vi "Calculate Torque.vi"() -> ()   [LabVIEW 2019]
doc: "This VI calculates the total torque resulting from two seperate force acting at two distinct moment arms. it uses a subvi to do the cross product.\n\nPK\nP3600"
uses:
  typedefs/torque vector.ctl
  P2 start/typedefs/moment arm vector.ctl
  P2 start/typedefs/force vector.ctl
panel:
  in  "Force B":T1={"Fx"=0.0, "Fy"=0.0, "Fz"=10.0}
  in  "Force A":T1={"Fx"=0.0, "Fy"=10.0, "Fz"=0.0}
  in  "Moment Arm B":T2={"Rx"=0.0, "Ry"=10.0, "Rz"=0.0}
  in  "Moment Arm A":T2={"Rx"=10.0, "Ry"=0.0, "Rz"=0.0}
  out "Resultant Torque":T3={"Nx"=100.0, "Ny"=0.0, "Nz"=100.0}
  # "Calculating Torques\n\nPK\nP3600"
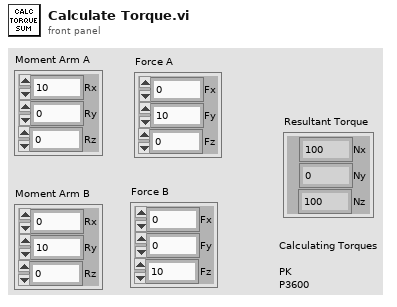
[diagram p1: front panel]
types:
  T1 = typedef "force vector.ctl" = cluster{"Fx":dbl, "Fy":dbl, "Fz":dbl}
  T2 = typedef "moment arm vector.ctl" = cluster{"Rx":dbl, "Ry":dbl, "Rz":dbl}
  T3 = typedef "torque vector.ctl" = cluster{"Nx":dbl, "Ny":dbl, "Nz":dbl}
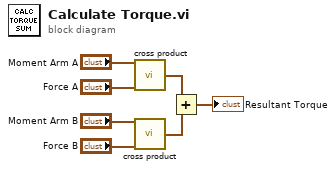
[diagram p0: block diagram]
diagram:
  n1 = call "cross product.vi"("Moment Arm"="Moment Arm A", "Force"="Force A") -> ("Torque"=w3:T3)  [unwired: 13 in]
  n2 = call "cross product.vi"("Moment Arm"="Moment Arm B", "Force"="Force B") -> ("Torque"=w2:T3)  [unwired: 13 in]
  n3 = Add(x=w3, y=w2) -> (x+y=→"Resultant Torque":T3)
